vi "IntakeNumbToState.vi"(11 "StateNumber":dbl) -> (3 "Intake_State":T1)   [LabVIEW 2023]
uses:
  IntakeState.ctl
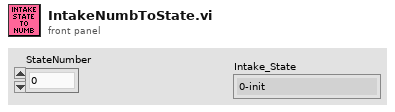
[diagram p1: front panel]
types:
  T1 = typedef "IntakeState.ctl" = enum16{"0-init", "1-cancel", "2-wait-for-cmd", "3-intake-check-for-note", "4-intake-start-intake", "5-intake-have-note-yet", "6-intake-stop-motor", "7-spit-out", "8-feed-note-to-shooter"}
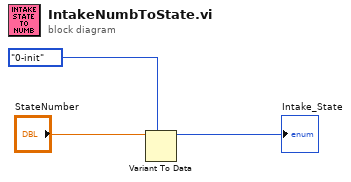
[diagram p0: block diagram]
diagram:
  n1 = Variant To Data(type=IntakeState."0-init" ("Intake_State"), Variant="StateNumber") -> (data=→"Intake_State":T1)  [unwired: 1 in, 1 out]
